vi "Export Profile.vi"(8 "error in (no error)":errorcluster, 9 "Password":string, 10 "SSID":string, 11 "XML path in":path) -> (0 "error out":errorcluster, 2 "Feedback":string, 3 "XML path out":path)   [LabVIEW 2017]
doc: "Saves WLAN profiles as XML files to the specified location."
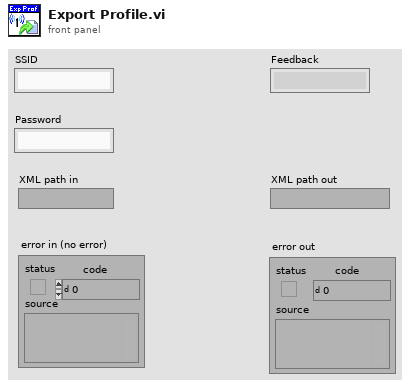
[diagram p1: front panel]
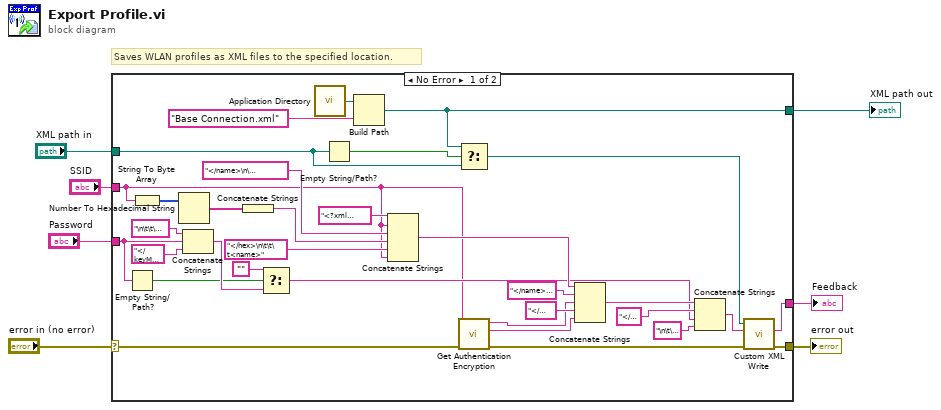
[diagram p0: block diagram]
diagram:
  # "Saves WLAN profiles as XML files to the specified location."
  n1 = case shown="No Error" "error in (no error)" {
    selector: "error in (no error)" -> [w8 w41]
    tunnel: [w19 w41] -> w6
    tunnel: "SSID" -> [w10 _]
    tunnel: "Password" -> [w12 _]
    tunnel: [w18 _] -> w3
    tunnel: "XML path in" -> [w15 _]
    tunnel: [w9 _] -> w1
    frame No Error {
      n2 = Empty String/Path?(string/path=w12) -> (empty?=w11:bool)
      n3 = String To Byte Array(string=w10) -> (unsigned byte array=w24:u8[])
      n4 = Number To Hexadecimal String(2:w24) -> (0:w23:string[])  [unwired: 1 in]
      n5 = Concatenate Strings("\n\t\t\t<sharedKey>\n\t\t\t\t<keyType>passPhrase</keyType>\n\t\t\t\t<protected>false</protected>\n\t\t\t\t<keyMaterial>" ("string"), w12, "</keyMaterial>\n\t\t\t</sharedKey>" ("string")) -> (w29:string)
      n6 = Concatenate Strings(w23) -> (w22:string)
      n7 = Select(t="", s=w11, f=w29) -> (s? t:f=w28:string)
      n8 = call <vilib>:"Application Directory.vi"() -> ("Application Directory"=w40:path)
      n9 = Empty String/Path?(string/path=w15) -> (empty?=w16:bool)
      n10 = Build Path(base path=w40, name or relative path="Base Connection.xml") -> (appended path=w18:path)
      n11 = Concatenate Strings("<?xml version=\"1.0\"?>\n<WLANProfile xmlns=\"http://www.microsoft.com/networking/WLAN/profile/v1\">\n\t<name>" ("string"), w10, "</name>\n\t<SSIDConfig>\n\t\t<SSID>\n\t\t\t<hex>" ("string"), w22, "</hex>\n\t\t\t<name>" ("string"), w10) -> (w37:string)
      n12 = Select(t=w18, s=w16, f=w15) -> (s? t:f=w17:path)
      n13 = call "Get Authentication Encryption.vi"("error in (no error)"=w8, "SSID"=w10) -> ("error out"=w20:errorcluster, "Encryption"=w34:string, "Authentication"=w31:string)  [unwired: 7 in]
      n14 = Concatenate Strings(w37, "</name>\n\t\t</SSID>\n\t</SSIDConfig>\n\t<connectionType>ESS</connectionType>\n\t<connectionMode>auto</connectionMode>\n\t<MSM>\n\t\t<security>\n\t\t\t<authEncryption>\n\t\t\t\t<authentication>" ("string"), w31, "</authentication>\n\t\t\t\t<encryption>" ("string"), w34) -> (w33:string)
      n15 = Concatenate Strings(w33, "</encryption>\n\t\t\t\t<useOneX>false</useOneX>\n\t\t\t</authEncryption>" ("string"), w28, "\n\t\t</security>\n\t</MSM>\n</WLANProfile>\n" ("string")) -> (w21:string)
      n16 = call "Custom XML Write.vi"("error in (no error)"=w20, "XML Input"=w21, "XML File Path"=w17) -> ("error out"=w19:errorcluster, "XML String"=w9:string)  [unwired: 6 in, 1 out]
    }
    frame Error {
    }
  }
  "error out" <- w6
  "XML path out" <- w3
  "Feedback" <- w1
